vi "Island Watch.vi"(8 "error in (no error)":errorcluster, 10 "Frequency Control":refnum<class "Message Enqueuer.lvclass">, 11 "IED in":refnum<class "IED.lvclass">) -> (0 "error out":errorcluster, 3 "IED out":refnum<class "IED.lvclass">)   [LabVIEW 2015, in "IED Actor.lvlib" / "IED.lvclass"]
uses:
  IED.lvclass
  <vilib>/ActorFramework/Message Enqueuer/Message Enqueuer.lvclass
  Island Watch Actor/Island Watch/Island Watch.lvclass
  IED.lvclass/IED.ctl
  <vilib>/ActorFramework/Actor/Actor.lvclass
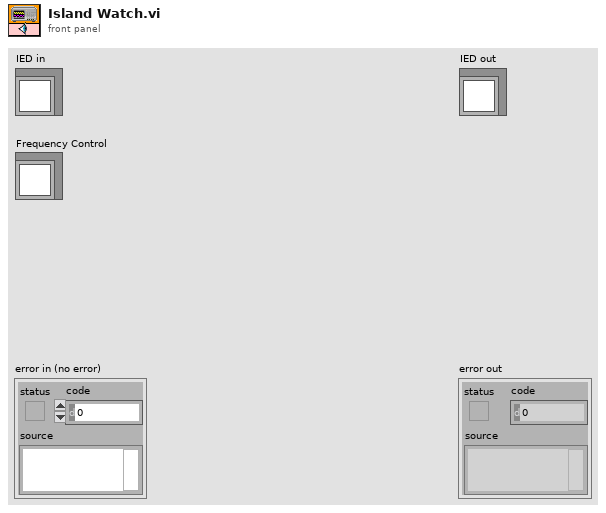
[diagram p1: front panel]
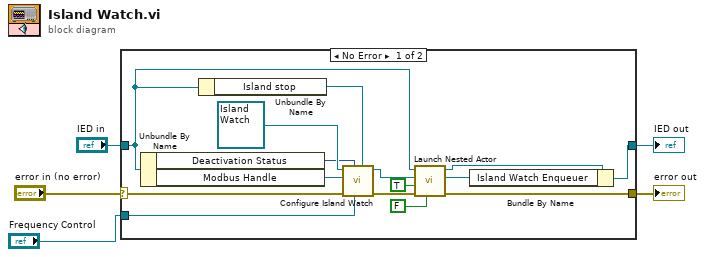
[diagram p0: block diagram]
diagram:
  n1 = case shown="No Error" "error in (no error)" {
    selector: "error in (no error)" -> [w18 w22]
    tunnel: [w13 w22] -> w4
    tunnel: [w11 w21] -> w2
    tunnel: "IED in" -> [w9 w21]
    tunnel: "Frequency Control" -> [w16 _]
    frame No Error {
      n2 = Unbundle By Name(w9) -> ("Deactivation Status"=w17:u16, "Modbus Handle"=w12:refnum<class "Modbus Master.lvclass">)
      n3 = Unbundle By Name(w9) -> ("Island stop"=w8:refnum<notifier>)
      n4 = call "Configure Island Watch.vi"("Island stop notifier"=w8, "Frequency Control"=w16, "Register"=w17, "error in (no error)"=w18, "Modbus Handle"=w12, "Island Watch in"=refnum<class "Island Watch.lvclass"> refnum ("Island Watch Actor.lvlib:Island Watch.lvclass")) -> ("error out"=w14:errorcluster, "Island Watch out"=w15:refnum<class "Island Watch.lvclass">)  [unwired: 4 in]
      n5 = call <vilib>:"Launch Nested Actor.vi"("Open Actor Core front panel? (F)"=FALSE, "error in (no error)"=w14, "Auto-stop? (T)"=TRUE, "Nested Actor"=w15, "Caller Actor in"=w9) -> ("error out"=w13:errorcluster, "Nested Actor's Enqueuer"=w10:refnum<class "Message Enqueuer.lvclass">, "Caller Actor out"=w20:refnum<class "IED.lvclass">)  [unwired: 4 in]
      n6 = Bundle By Name(cluster=w20, "Island Watch Enqueuer"=w10) -> (w11:refnum<class "IED.lvclass">)
    }
    frame Error {
    }
  }
  "error out" <- w4
  "IED out" <- w2
